vi "Operator Login Dialog.vi"() -> (3 "Logged In?":bool)   [LabVIEW 2020]
doc: "Use this template to create a dialog box with event handling."
uses:
  System.DirectoryServices.AccountManagement
panel:
  in  "contextType":i32(ring) items=["Machine", "Domain", "ApplicationDirectory"]
  out "Groups":string[](array[string])
  out "Operator Name":string
  in  "Password":string
  in  "Operator Name":string
  in  "Cancel":bool
  in  "Login":bool
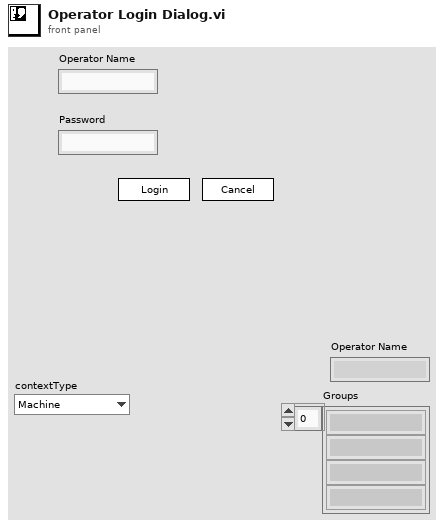
[diagram p1: front panel]
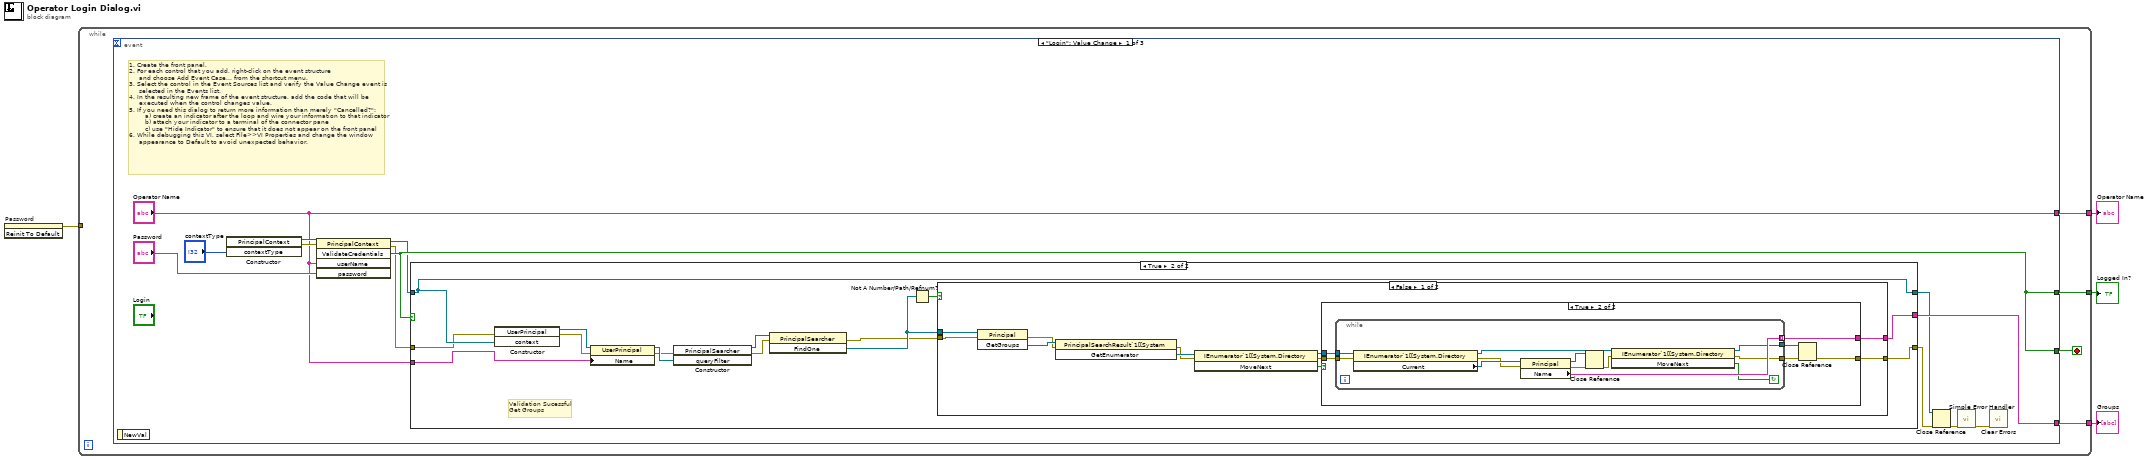
[diagram p0: block diagram]
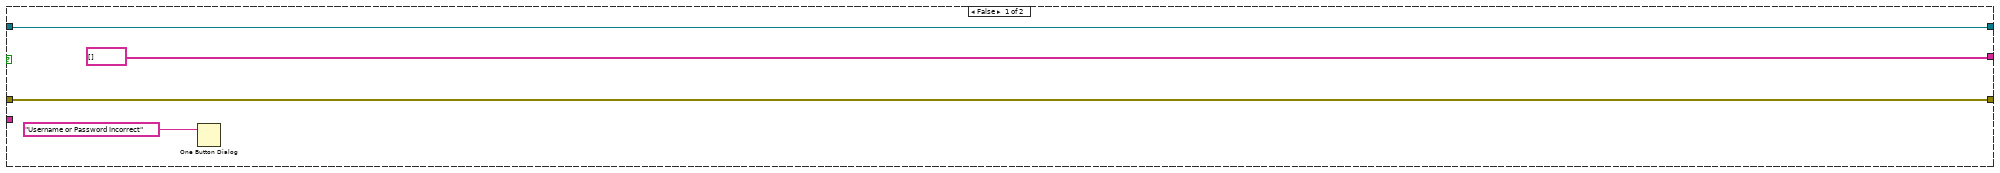
[diagram p2: hidden frame]
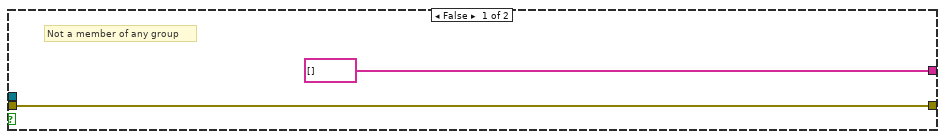
[diagram p3: hidden frame]
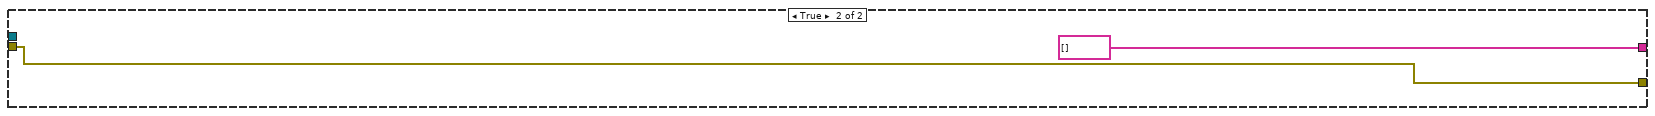
[diagram p4: hidden frame]
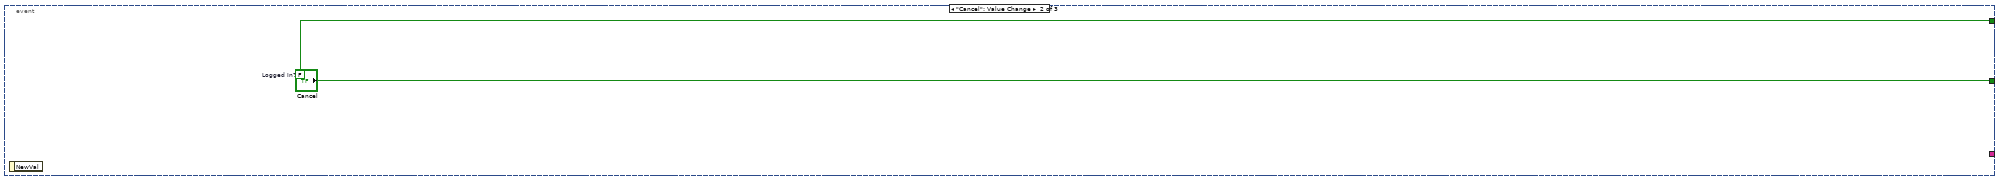
[diagram p5: hidden frame]
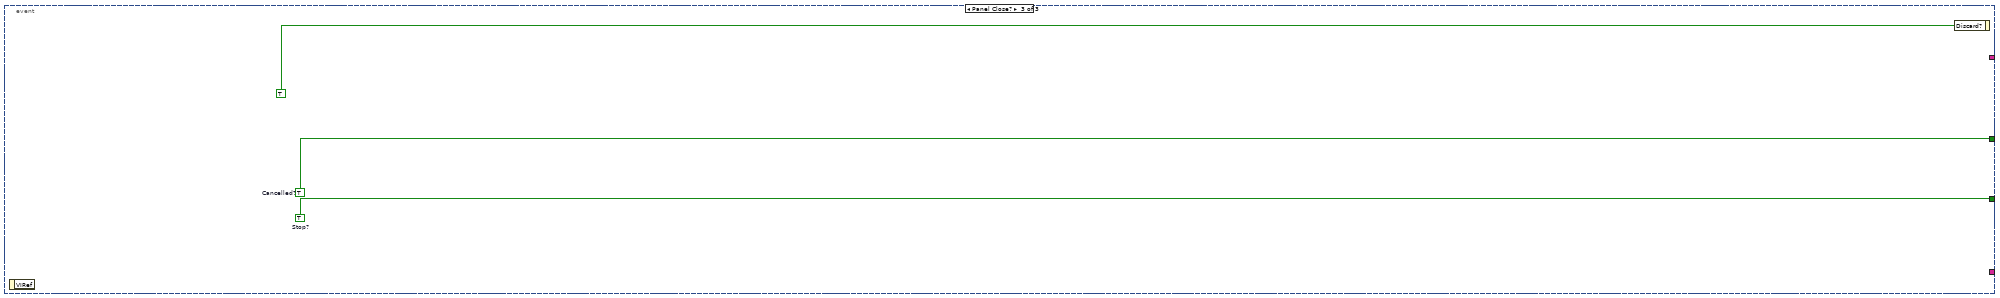
[diagram p6: hidden frame]
diagram:
  n1 = invoke on="Password" class="Str" method="Reinit To Default"() -> (error out=w1:errorcluster)  [unwired: 3 in, 2 out]
  n2 = while {
    tunnel: [w7] -> w4
    tunnel: [w6] -> w3
    tunnel: [w5] -> w2
    tunnel: w1 -> [_]
    stop <- w8 stop-if-true
    n3 = event shown="[0] \"Login\": Value Change" {
      selector: _ -> [_ _ _]
      dyn-events: _ -> [_ _ _]
      timeout: _ -> [_ _ _]
      tunnel: [w17 "Cancel" w76] -> w8
      tunnel: [w17 w74 w75] -> w7
      tunnel: ["Operator Name" _ _] -> w6
      tunnel: [w14 _ _] -> w5
      event "Login": Value Change {
        # "1. Create the front panel.\n2. For each control that you add, right-click on the event structure \n     and choose Add Event Case... from the shortcut menu.\n3. Select the control in the Event Sources list and verify the Value Change event is \n     selected in the Events list.\n4. In the resulting new frame of the event structure, add the code that will be \n     executed when the control changes value.\n5. If you need this dialog to return more information than merely \"Cancelled?\":\n        a) create an indicator after the loop and wire your information to that indicator\n        b) attach your indicator to a terminal of the connector pane\n        c) use \"Hide Indicator\" to ensure that it does not appear on the front panel\n6. While debugging this VI, select File>>VI Properties and change the window \n     appearance to Default to avoid unexpected behavior."
        n4 = event-data() -> ()  [unwired: 1 in, 1 out]
        n5 = constructor class="PrincipalContext"("contextType"="contextType") -> (reference out=w19:refnum<k24>, error out=w20:errorcluster)  [unwired: 3 in, 2 out]
        n6 = invoke class="PrincipalContext" method="ValidateCredentials"(reference=w19, error in=w20, "userName"="Operator Name", "password"="Password") -> (reference out=w13:refnum<k24>, error out=w12:errorcluster, "ValidateCredentials"=w17:bool)  [unwired: 1 in, 2 out]
        n7 = case shown="True" w17 {
          tunnel: [string[] [] ("Groups") w35] -> w14
          tunnel: w13 -> [w23 w39]
          tunnel: w12 -> [w24 w32]
          tunnel: [w24 w34] -> w11
          tunnel: [w23 w39] -> w10
          tunnel: "Operator Name" -> [_ w38]
          frame False {
            n8 = One Button Dialog(message="Username or Password Incorrect") -> ()  [unwired: 1 in, 1 out]
          }
          frame True {
            # "Validation Sucessful\nGet Groups"
            n9 = constructor class="UserPrincipal"(error in=w32, "context"=w39) -> (reference out=w31:refnum<k24>, error out=w30:errorcluster)  [unwired: 2 in, 2 out]
            n10 = property class="UserPrincipal"(reference=w31, error in=w30, "Name"=w38) -> (reference out=w29:refnum<k24>, error out=w28:errorcluster)
            n11 = constructor class="PrincipalSearcher"(error in=w28, "queryFilter"=w29) -> (reference out=w26:refnum<k24>, error out=w27:errorcluster)  [unwired: 2 in, 2 out]
            n12 = invoke class="PrincipalSearcher" method="FindOne"(reference=w26, error in=w27) -> (error out=w33:errorcluster, "FindOne"=w37:refnum<k24>)  [unwired: 1 in, 1 out]
            n13 = Not A Number/Path/Refnum?(number/path/refnum=w37) -> (NaN/Path/Refnum?=w36:bool)
            n14 = case shown="False" w36 {
              tunnel: w37 -> [w50 _]
              tunnel: [w44 string[] [] ("Groups")] -> w35
              tunnel: [w42 w72] -> w34
              tunnel: w33 -> [w41 w72]
              frame False {
                n15 = invoke class="Principal" method="GetGroups"(reference=w50, error in=w41) -> (error out=w40:errorcluster, "rvices.AccountManagement, Version=0.0.0.0, Culture=neutral, PublicKeyToken=b77a5c561934e089\tGetGroups"=w49:refnum<k24>)  [unwired: 1 in, 1 out]
                n16 = invoke class="PrincipalSearchResult`1[[System" method="GetEnumerator"(reference=w49, error in=w40) -> (error out=w47:errorcluster, "GetEnumerator"=w48:refnum<k24>)  [unwired: 1 in, 1 out]
                n17 = invoke class="IEnumerator`1[[System.Directory" method="MoveNext"(reference=w48, error in=w47) -> (reference out=w46:refnum<k24>, error out=w43:errorcluster, "MoveNext"=w45:bool)  [unwired: 1 in]
                n18 = case shown="True" w45 {
                  tunnel: w46 -> [_ w58]
                  tunnel: [string[] [] ("Groups") w56] -> w44
                  tunnel: w43 -> [w51 w57]
                  tunnel: [w51 w53] -> w42
                  frame False {
                    # "Not a member of any group"
                  }
                  frame True {
                    n19 = while {
                      tunnel: w58 -> [w70]
                      tunnel: w57 -> [w69]
                      tunnel: [w65] -> w56 mode=indexing
                      tunnel: [w63] -> w55
                      tunnel: [w59] -> w54
                      stop <- w64 continue-if-true
                      n20 = property class="IEnumerator`1[[System.Directory"(reference=w70, error in=w69) -> (reference out=w66:refnum<k24>, error out=w67:errorcluster, "Current"=w68:refnum<k24>)
                      n21 = property class="Principal"(reference=w68, error in=w67) -> (reference out=w62:refnum<k24>, error out=w61:errorcluster, "Name"=w65:string)
                      n22 = Close Reference(reference=w62, error in (no error)=w61) -> (error out=w60:errorcluster)
                      n23 = invoke class="IEnumerator`1[[System.Directory" method="MoveNext"(reference=w66, error in=w60) -> (reference out=w59:refnum<k24>, error out=w63:errorcluster, "MoveNext"=w64:bool)  [unwired: 1 in]
                    }
                    n24 = Close Reference(reference=w54, error in (no error)=w55) -> (error out=w53:errorcluster)
                  }
                }
              }
              frame True {
              }
            }
          }
        }
        n25 = Close Reference(reference=w10, error in (no error)=w11) -> (error out=w16:errorcluster)
        n26 = call <vilib>:"Simple Error Handler.vi"("error in (no error)"=w16) -> ("error out"=w15:errorcluster)  [unwired: 4 in, 4 out]
        n27 = call <vilib>:"Clear Errors.vi"("error in (no error)"=w15) -> ()  [unwired: 5 in, 2 out]
      }
      event "Cancel": Value Change {
        w74 = FALSE  # Logged In?
        n28 = event-data() -> ()  [unwired: 1 in, 1 out]
      }
      event Panel Close? {
        w75 = TRUE  # Cancelled?
        w76 = TRUE  # Stop?
        n29 = event-data() -> ()  [unwired: 1 in, 1 out]
        n30 = event-data("Discard?"=TRUE) -> ()  [unwired: 1 in, 1 out]
      }
    }
  }
  "Logged In?" <- w4
  "Operator Name" <- w3
  "Groups" <- w2
